vi "Player Info.vi"(11 "Lone Wolf in":refnum<class "Cautious Wolf.lvclass">) -> (0 "Defeat Speech":string, 1 "Victory Speech":string, 2 "Name":string, 3 "Lone Wolf out":refnum<class "Cautious Wolf.lvclass">)   [LabVIEW 2020, in "Cautious Wolf.lvclass"]
uses:
  Cautious Wolf.lvclass
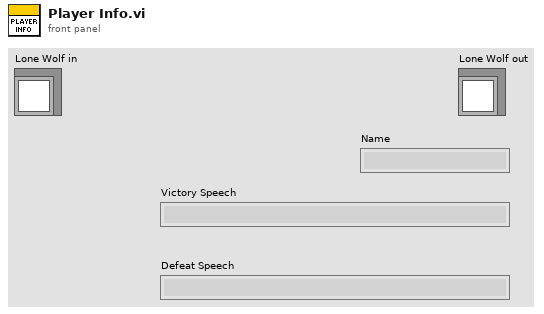
[diagram p1: front panel]
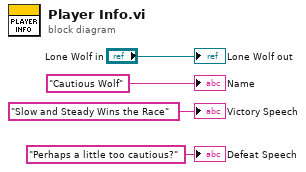
[diagram p0: block diagram]
diagram:
  "Lone Wolf out" <- "Lone Wolf in"
  "Name" <- "Cautious Wolf" ("Name")
  "Victory Speech" <- "Slow and Steady Wins the Race" ("Victory Speech")
  "Defeat Speech" <- "Perhaps a little too cautious?" ("Defeat Speech")
